vi "Write Numeric.vi"(8 "error in (no error)":errorcluster, 10 "Numeric":dbl, 11 "ExampleClass in":refnum<class "ExampleClass.lvclass">) -> (0 "error out":errorcluster, 3 "ExampleClass out":refnum<class "ExampleClass.lvclass">)   [LabVIEW 2014, in "ExampleClass.lvclass"]
uses:
  ExampleClass.lvclass
  ExampleClass.lvclass/ExampleClass.ctl
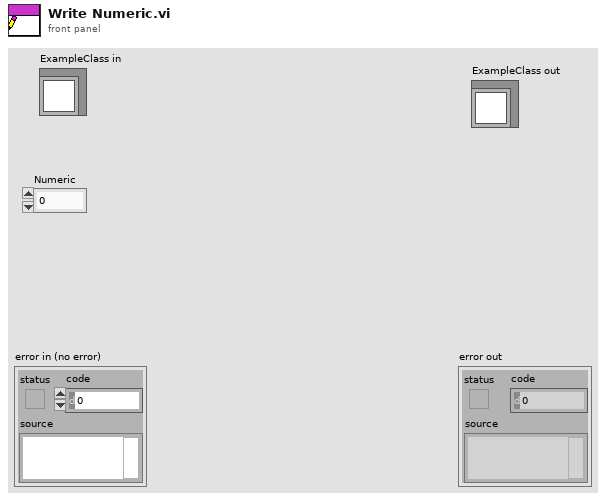
[diagram p1: front panel]
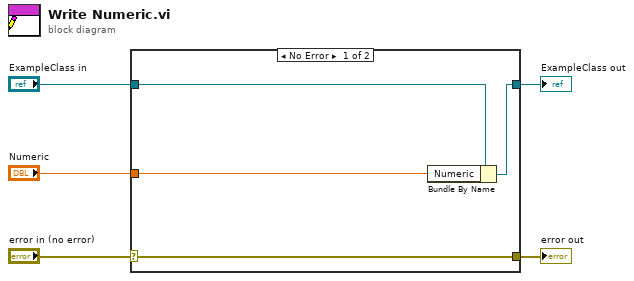
[diagram p0: block diagram]
diagram:
  n1 = case shown="No Error" "error in (no error)" {
    selector: "error in (no error)" -> [w9 w10]
    tunnel: [w9 w10] -> w4
    tunnel: [w7 w11] -> w2
    tunnel: "ExampleClass in" -> [w8 w11]
    tunnel: "Numeric" -> [w6 _]
    frame No Error {
      n2 = Bundle By Name(cluster=w8, "Numeric"=w6) -> (w7:refnum<class "ExampleClass.lvclass">)
    }
    frame Error {
    }
  }
  "error out" <- w4
  "ExampleClass out" <- w2
